vi "Update.vi"(11 "服务器信息":T1={"host"="27.154.58.30", "port"=8020, "user"="std", "password"="std23506", "远端地址"="/微站/室外总磷总氮高压过滤无主板新电路板/一体化微型水质监测站.exe"}) -> ()   [LabVIEW 2016, in "数据传输系统-03.lvlib" / "update.lvlib"]
uses:
  update.lvlib
panel:
  out "已下载大小":sgl format="%.2f MB"
  out "滑动杆":dbl(slide) scale=0.0..100.0
  in  "取消按钮":bool
  out "last status string":string caption="最近状态字符串"
  out "command":string caption="命令"
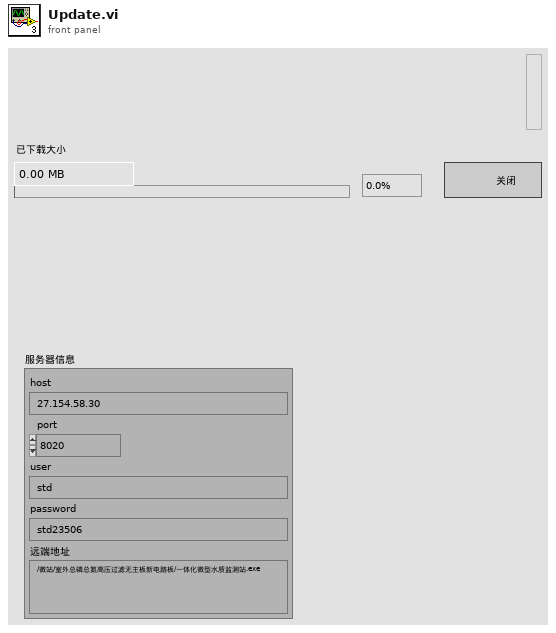
[diagram p1: front panel]
types:
  T1 = cluster{"host":string, "port":u16, "user":string, "password":string, "远端地址":string}
  T2 = cluster{"command":string, "last status string":string, "process":dbl}
  T3 = enum32{"Bad", "Idle", "Run top level", "Running"}
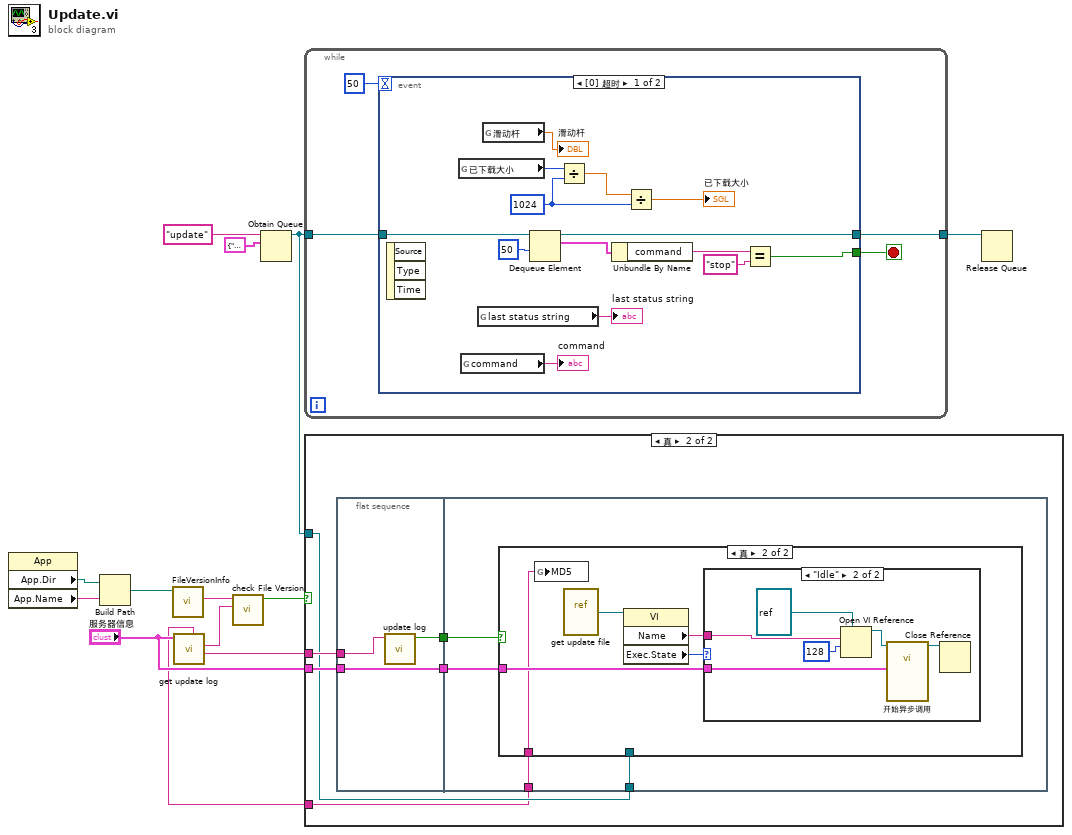
[diagram p0: block diagram]
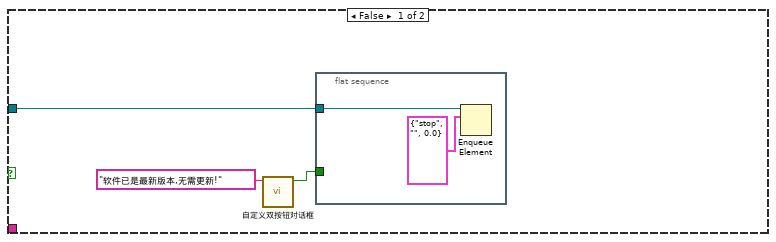
[diagram p2: hidden frame]
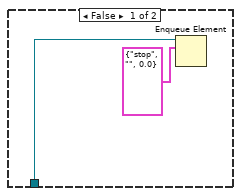
[diagram p3: hidden frame]
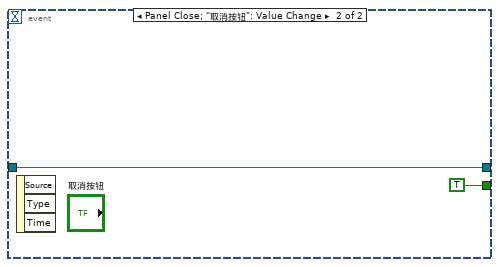
[diagram p5: hidden frame]
diagram:
  n1 = property class="App"() -> ("App.Dir"=w8:path, "App.Name"=w7:string)  [unwired: 2 in, 2 out]
  n2 = Build Path(base path=w8, name or relative path=w7) -> (appended path=w6:path)
  n3 = call <vilib>:"FileVersionInfo.vi"("Application Path in"=w6) -> ("File Version Info"=w2:string)  [unwired: 7 in, 3 out]
  n4 = call "get update log.vi"("服务器信息"="服务器信息") -> ("部分更新日志"=w4:string, "remote File Version"=w9:string, "MD5"=w1:string)  [unwired: 6 in, 2 out]
  n5 = call "check File Version.vi"("remote File Version Info"=w9, "Local File Version Info"=w2) -> ("new?"=w3:bool)  [unwired: 9 in]
  n6 = Obtain Queue(name (unnamed)="update" ("名称（未命名）"), element data type=T2 {"command"="", "last status string"="", "process"=0.0}) -> (queue out=w5:refnum<queue>)  [unwired: 3 in, 2 out]
  n7 = while {
    tunnel: w5 -> [w15]
    tunnel: [w14] -> w12
    stop <- w16 stop-if-true
    n8 = event shown="[0] 超时" {
      selector: _ -> [_ _]
      dyn-events: _ -> [_ _]
      timeout: 50 -> [_ _]
      tunnel: [w26 TRUE] -> w16
      tunnel: w15 -> [w31 w32]
      tunnel: [w29 w32] -> w14
      event Timeout {
        w19 = i64 1024 ("y")
        n9 = event-data() -> ()  [unwired: 1 in, 3 out]
        n10 = global read "更新全局变量.vi" "已下载大小"() -> (w21:i64)
        n11 = global read "更新全局变量.vi" "command"() -> (→"command":string)
        n12 = global read "更新全局变量.vi" "last status string"() -> (→"last status string":string)
        n13 = global read "更新全局变量.vi" "滑动杆"() -> (→"滑动杆":dbl)
        n14 = Dequeue Element(queue=w31, timeout in ms (-1)=50 ("超时毫秒(-1)")) -> (queue out=w29:refnum<queue>, element=w30:T2)  [unwired: 1 in, 2 out]
        n15 = Divide(x=w21, y=w19) -> (x/y=w20:dbl)
        n16 = Unbundle By Name(w30) -> ("command"=w28:string)
        n17 = Divide(x=w20, y=w19) -> (x/y=→"已下载大小":dbl)
        n18 = Equal?(x=w28, y="stop") -> (x = y?=w26:bool)
      }
      event Panel Close; "取消按钮": Value Change {
        n19 = event-data() -> ()  [unwired: 1 in, 3 out]
      }
    }
  }
  n20 = case shown="真" w3 {
    tunnel: "服务器信息" -> [_ w44]
    tunnel: w4 -> [_ w42]
    tunnel: w5 -> [w36 w40]
    tunnel: w1 -> [_ w39]
    frame False {
      n21 = call "自定义双按钮对话框.vi"("消息"="软件已是最新版本,无需更新!") -> ("输出"=w34:bool)  [unwired: 10 in]
      n22 = flat-sequence {
        tunnel: w36 -> [w38]
        tunnel: w34 -> [_]
        frame #0 {
          n23 = Enqueue Element(queue=w38, element=T2 {"command"="stop", "last status string"="", "process"=0.0} ("元素")) -> ()  [unwired: 2 in, 3 out]
        }
      }
    }
    frame True {
      n24 = flat-sequence {
        tunnel: w44 -> [w47]
        tunnel: [w47] -> w43
        tunnel: w42 -> [w46]
        tunnel: [w45] -> w41
        tunnel: w43 -> [w51]
        tunnel: w41 -> [w50]
        tunnel: w40 -> [w49]
        tunnel: w39 -> [w48]
        frame #0 {
          n25 = call "update log.vi"("更新记录"=w46) -> ("check"=w45:bool)  [unwired: 10 in]
        }
        frame #1 {
          n26 = case shown="真" w50 {
            tunnel: w51 -> [_ w55]
            tunnel: w49 -> [w52 _]
            tunnel: w48 -> [_ w54]
            frame False {
              n27 = Enqueue Element(queue=w52, element=T2 {"command"="stop", "last status string"="", "process"=0.0} ("元素")) -> ()  [unwired: 2 in, 3 out]
            }
            frame True {
              n28 = global write "更新全局变量.vi" "MD5"(w54) -> ()
              n29 = vi-ref "get update file.vi"() -> (w58:refnum<vi>)
              n30 = property class="VI"(reference=w58) -> ("Name"=w57:string, "Exec.State"=w56:T3)  [unwired: 1 in, 2 out]
              n31 = case shown="\"Idle\"" w56 {
                tunnel: w57 -> [_ w64]
                tunnel: w55 -> [_ w60]
                frame "Bad", Default {
                }
                frame "Idle" {
                  n32 = Open VI Reference(type specifier VI Refnum (for type only)=refnum<vi> refnum, vi path=w64, options=128 ("选项")) -> (vi reference=w61:refnum<vi>)  [unwired: 3 in, 1 out]
                  n33 = call-by-ref "开始异步调用"(reference=w61, "服务器信息"=w60) -> (reference out=w62:refnum<vi>)  [unwired: 12 in, 1 out]
                  n34 = Close Reference(reference=w62) -> ()  [unwired: 1 in, 1 out]
                }
              }
            }
          }
        }
      }
    }
  }
  n35 = Release Queue(queue=w12) -> ()  [unwired: 2 in, 3 out]
